vi "FGV-MassData.vi"(6 "Operation":T1, 8 "Error in":errorcluster caption="Error in (no error)", 9 "size":i32, 10 "Start":i32, 11 "Data in":dbl[](array[numeric])) -> (0 "Error out":errorcluster, 1 "Active Read Oper":T2, 2 "Active Write Oper":T2, 3 "Data out":dbl[](array[numeric]))   [LabVIEW 2020, in "JKISM++ Array Parameter Support.lvlib"]
uses:
  JKISM++ Array Parameter Support.lvlib
  Def-MassDataOper-Status.ctl
  Operation-FGV-MassData.ctl
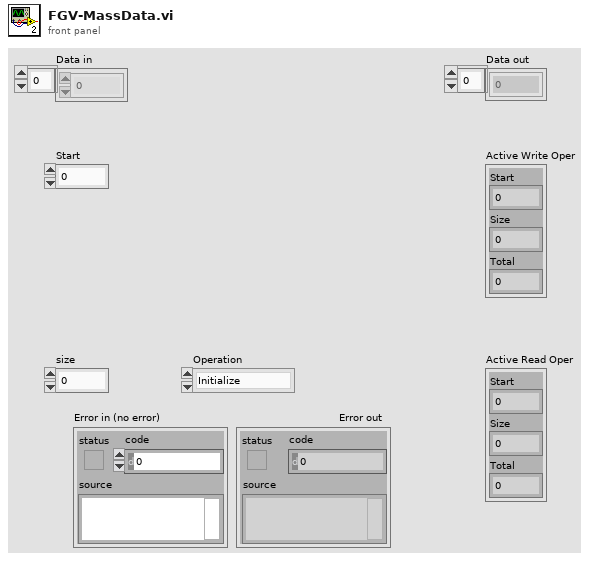
[diagram p1: front panel]
types:
  T1 = typedef "JKISM++ Array Parameter Support.lvlib/Operation-FGV-MassData.ctl" = enum16{"Initialize", "Read", "Write", "Status", "Release"}
  T2 = typedef "JKISM++ Array Parameter Support.lvlib/Def-MassDataOper-Status.ctl" = cluster{"Start":i32, "Size":i32, "Total":i32}
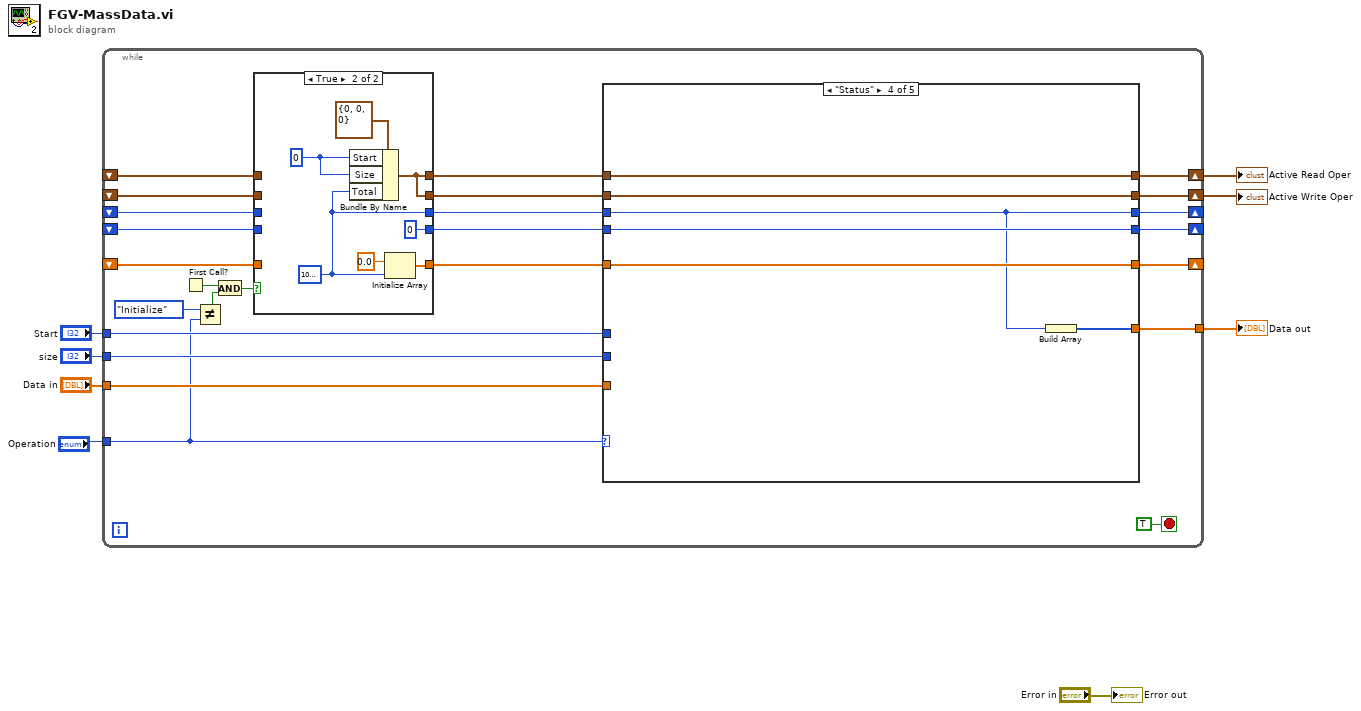
[diagram p0: block diagram]
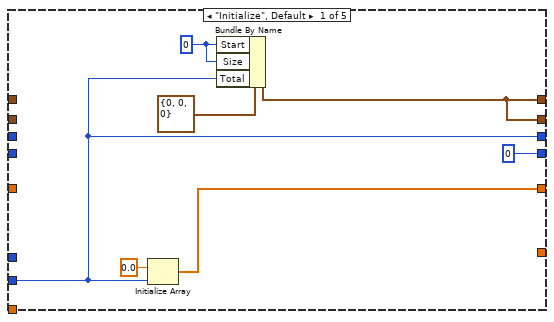
[diagram p3: hidden frame]
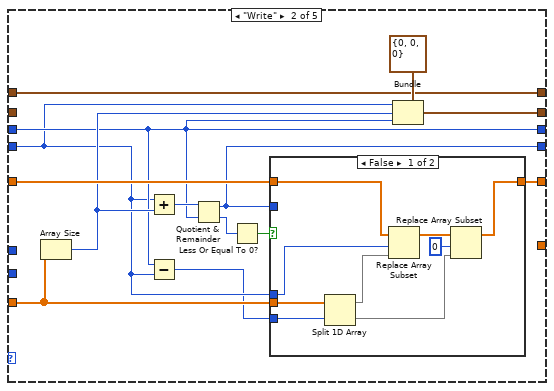
[diagram p4: hidden frame]
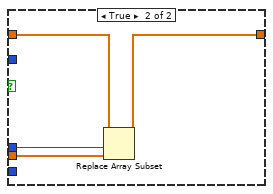
[diagram p5: hidden frame]
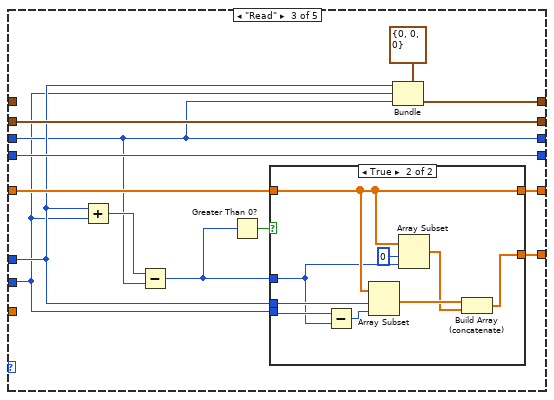
[diagram p6: hidden frame]
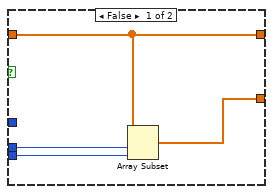
[diagram p7: hidden frame]
diagram:
  n1 = while {
    tunnel: "Operation" -> [w21]
    shift-right: [w32] -> _
    shift-left: _ -> [w9]
    tunnel: "Start" -> [w31]
    tunnel: "size" -> [w30]
    tunnel: [w29] -> w5
    tunnel: "Data in" -> [w28]
    shift-right: [w27] -> _
    shift-left: _ -> [w12]
    shift-right: [w26] -> w2
    shift-left: _ -> [w15]
    shift-right: [w25] -> w3
    shift-left: _ -> [w18]
    shift-right: [w24] -> _
    shift-left: _ -> [w11]
    stop <- TRUE stop-if-true
    n2 = First Call?() -> (First Call?: T/F=w23:bool)
    n3 = Not Equal?(x=Operation-FGV-MassData."Initialize", y=w21) -> (x != y?=w22:bool)
    n4 = And(x=w23, y=w22) -> (x .and. y?=w19:bool)
    n5 = case shown="True" w19 {
      tunnel: w18 -> [w38 _]
      tunnel: [w38 w40] -> w17
      tunnel: [w37 w40] -> w16
      tunnel: w15 -> [w37 _]
      tunnel: [w36 w41] -> w14
      tunnel: [w35 0 ("Start")] -> w13
      tunnel: w12 -> [w36 _]
      tunnel: w11 -> [w35 _]
      tunnel: [w34 w44] -> w10
      tunnel: w9 -> [w34 _]
      frame False {
      }
      frame True {
        w42 = 0 ("Start")
        w41 = 1000000
        n6 = Bundle By Name(cluster=T2 {"Start"=0, "Size"=0, "Total"=0} ("Cache Status"), "Start"=w42, "Size"=w42, "Total"=w41) -> (w40:T2)
        n7 = Initialize Array(0.0, w41) -> (w44:dbl[])
      }
    }
    n8 = case shown="\"Status\"" w21 {
      tunnel: [w48 w65 w91 w111 w116] -> w32
      tunnel: w10 -> [_ w66 w92 w111 w116]
      tunnel: w31 -> [_ _ w85 _ _]
      tunnel: w30 -> [w49 _ w81 _ _]
      tunnel: [_ _ w80 w107 _] -> w29
      tunnel: w28 -> [_ w64 _ _ _]
      tunnel: [w49 w55 w83 w106 w115] -> w27
      tunnel: w14 -> [_ w55 w83 w106 w115]
      tunnel: [w51 w62 w87 w110 w114] -> w26
      tunnel: w16 -> [_ _ w87 w110 w114]
      tunnel: [w51 w61 w88 w109 w113] -> w25
      tunnel: w17 -> [_ w61 _ w109 w113]
      tunnel: w13 -> [_ w54 w86 w108 w112]
      tunnel: [0 ("Start") w57 w86 w108 w112] -> w24
      frame "Initialize", Default {
        w52 = 0 ("Start")
        n9 = Initialize Array(0.0, w49) -> (w48:dbl[])
        n10 = Bundle By Name(cluster=T2 {"Start"=0, "Size"=0, "Total"=0} ("Cache Status"), "Start"=w52, "Size"=w52, "Total"=w49) -> (w51:T2)
      }
      frame "Write" {
        n11 = Array Size(array=w64) -> (size(s)=w56:i32)
        n12 = Add(x=w54, y=w56) -> (x+y=w60:i32)
        n13 = Subtract(x=w55, y=w54) -> (x-y=w53:i32)
        n14 = Quotient & Remainder(x=w60, y=w55) -> (x-y*floor(x/y)=w57:i32, floor(x/y)=w59:i32)
        n15 = Less Or Equal To 0?(x=w59) -> (x <= 0?=w58:bool)
        n16 = case shown="False" w58 {
          tunnel: w66 -> [w75 w79]
          tunnel: [w71 w78] -> w65
          tunnel: w64 -> [w73 w77]
          tunnel: w54 -> [w74 w76]
          tunnel: w57 -> [_ _]
          tunnel: w53 -> [w67 _]
          frame False {
            n17 = Split 1D Array(array=w73, index=w67) -> (first subarray=w68:dbl[], second subarray=w69:dbl[])
            n18 = Replace Array Subset(array=w75, new element=w68, index=w74) -> (w72:dbl[])
            n19 = Replace Array Subset(array=w72, new element=w69, index=0) -> (w71:dbl[])
          }
          frame True {
            n20 = Replace Array Subset(array=w79, new element=w77, index=w76) -> (w78:dbl[])
          }
        }
        n21 = Bundle(cluster=T2 {"Start"=0, "Size"=0, "Total"=0} ("Cache Status"), "Start"=w54, "Size"=w56, "Total"=w55) -> (w62:T2)
      }
      frame "Read" {
        n22 = Add(x=w85, y=w81) -> (x+y=w84:i32)
        n23 = Subtract(x=w84, y=w83) -> (x-y=w82:i32)
        n24 = Greater Than 0?(x=w82) -> (x > 0?=w89:bool)
        n25 = case shown="True" w89 {
          tunnel: w92 -> [w95 w105]
          tunnel: [w95 w105] -> w91
          tunnel: w85 -> [w96 w104]
          tunnel: w82 -> [_ w98]
          tunnel: w81 -> [w94 w99]
          tunnel: [w93 w100] -> w80
          frame False {
            n26 = Array Subset(array=w95, index=w96, length=w94) -> (w93:dbl[])
          }
          frame True {
            n27 = Subtract(x=w99, y=w98) -> (x-y=w97:i32)
            n28 = Array Subset(array=w105, index=w104, length=w97) -> (w102:dbl[])
            n29 = Array Subset(array=w105, index=0, length=w98) -> (w101:dbl[])
            n30 = Build Array (concatenate)(w102, w101) -> (w100:dbl[])
          }
        }
        n31 = Bundle(cluster=T2 {"Start"=0, "Size"=0, "Total"=0} ("Cache Status"), "Start"=w85, "Size"=w81, "Total"=w83) -> (w88:T2)
      }
      frame "Status" {
        n32 = Build Array(w106) -> (w107:i32[])
      }
      frame "Release" {
      }
    }
  }
  "Data out" <- w5
  "Active Read Oper" <- w3
  "Active Write Oper" <- w2
  "Error out" <- "Error in"
